vi "Pressures.vi"(7 "Pressure":dbl, 8 "Error In":errorcluster, 9 "File Name In":path, 10 "Interruption Time":dbl, 11 "Flow":dynamicdata(graph)) -> (0 "Error Out":errorcluster, 1 "File Name":path, 2 "Interruption Time":dbl format="%#.3g", 3 "SGP":dbl, 5 "PTP":dbl)   [LabVIEW 2013]
uses:
  Controls/Intervals.ctl
  <vilib>/Utility/miscctls.llb/LVCursorListTypeDef.ctl
  <vilib>/Waveform/WDTOps.llb/WDT Get XY Value DBL.vi
panel:
  in  "Cursor List":T1=[{"Name"="L", "Color"=9843450, "Style"=2, "Point Style"=1, "Name Visible"=FALSE, "Allow Drag"=TRUE, "Cursor Mode"=0, "Plot"=0, "Index"=0, "Position"={"X"=3.0, "Y"=0.0}, "X Scale"=0, "Y Scale"=0, "Watch Plots"=[], "Watch All Plots"=FALSE, "Plot Area"=0, "Label Offset"={"X"=0.0, "Y"=0.0}}, {"Name"="R", "Color"=681210, "Style"=2, "Point Style"=1, "Name Visible"=FALSE, "Allow Drag"=TRUE, "Cursor Mode"=0, "Plot"=0, "Index"=0, "Position"={"X"=3.5, "Y"=0.0}, "X Scale"=0, "Y Scale"=0, "Watch Plots"=[], "Watch All Plots"=FALSE, "Plot Area"=0, "Label Offset"={"X"=0.0, "Y"=0.0}}]
  out "Subset":dynamicdata(graph)
  out "Flow":dynamicdata(graph)
  in  "Interval (ms)":T2 items=["1000", "500", "330", "250", "150", "50"]
  in  "Fixed Length?":bool
  in  "Mark Flow":bool
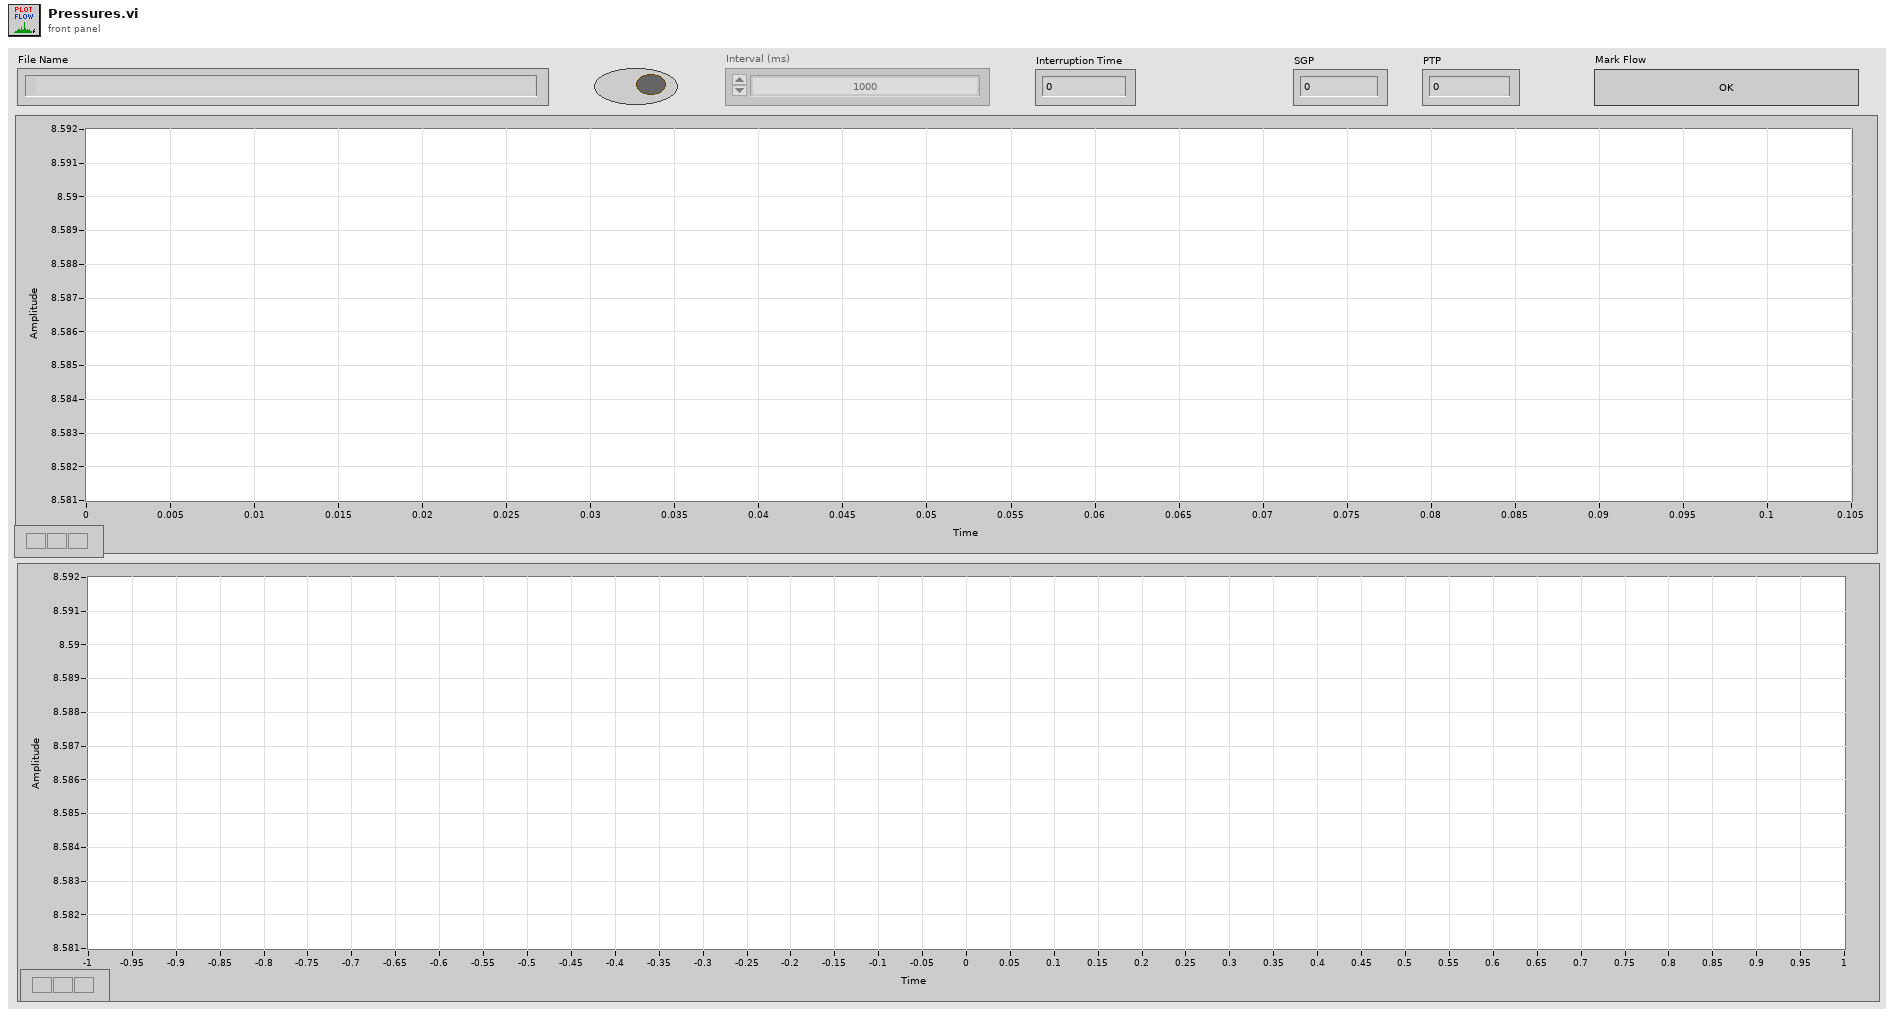
[diagram p1: front panel]
types:
  T1 = typedef "LVCursorListTypeDef.ctl" = cluster{"Name":string, "Color":u32, "Style":u8, "Point Style":u8, "Name Visible":bool, "Allow Drag":bool, "Cursor Mode":u32, "Plot":i32, "Index":i32, "Position":cluster{"X":dbl, "Y":dbl}, "X Scale":u32, "Y Scale":u32, "Watch Plots":i32[], "Watch All Plots":bool, "Plot Area":i32, "Label Offset":cluster{"X":dbl, "Y":dbl}}[]
  T2 = typedef "Intervals.ctl" = u16
  T3 = enum8{"Enabled", "Disabled", "Disabled and Grayed Out"}
  T4 = cluster{"Cursor List[0]":cluster{"Name":string, "Color":u32, "Style":u8, "Point Style":u8, "Name Visible":bool, "Allow Drag":bool, "Cursor Mode":u32, "Plot":i32, "Index":i32, "Position":cluster{"X":dbl, "Y":dbl}, "X Scale":u32, "Y Scale":u32, "Watch Plots":i32[], "Watch All Plots":bool, "Plot Area":i32, "Label Offset":cluster{"X":dbl, "Y":dbl}}, "Cursor List[1]":cluster{"Name":string, "Color":u32, "Style":u8, "Point Style":u8, "Name Visible":bool, "Allow Drag":bool, "Cursor Mode":u32, "Plot":i32, "Index":i32, "Position":cluster{"X":dbl, "Y":dbl}, "X Scale":u32, "Y Scale":u32, "Watch Plots":i32[], "Watch All Plots":bool, "Plot Area":i32, "Label Offset":cluster{"X":dbl, "Y":dbl}}, "Cursor List[2]":cluster{"Name":string, "Color":u32, "Style":u8, "Point Style":u8, "Name Visible":bool, "Allow Drag":bool, "Cursor Mode":u32, "Plot":i32, "Index":i32, "Position":cluster{"X":dbl, "Y":dbl}, "X Scale":u32, "Y Scale":u32, "Watch Plots":i32[], "Watch All Plots":bool, "Plot Area":i32, "Label Offset":cluster{"X":dbl, "Y":dbl}}, "Cursor List[3]":cluster{"Name":string, "Color":u32, "Style":u8, "Point Style":u8, "Name Visible":bool, "Allow Drag":bool, "Cursor Mode":u32, "Plot":i32, "Index":i32, "Position":cluster{"X":dbl, "Y":dbl}, "X Scale":u32, "Y Scale":u32, "Watch Plots":i32[], "Watch All Plots":bool, "Plot Area":i32, "Label Offset":cluster{"X":dbl, "Y":dbl}}, "Cursor List[4]":cluster{"Name":string, "Color":u32, "Style":u8, "Point Style":u8, "Name Visible":bool, "Allow Drag":bool, "Cursor Mode":u32, "Plot":i32, "Index":i32, "Position":cluster{"X":dbl, "Y":dbl}, "X Scale":u32, "Y Scale":u32, "Watch Plots":i32[], "Watch All Plots":bool, "Plot Area":i32, "Label Offset":cluster{"X":dbl, "Y":dbl}}, "Cursor List[5]":cluster{"Name":string, "Color":u32, "Style":u8, "Point Style":u8, "Name Visible":bool, "Allow Drag":bool, "Cursor Mode":u32, "Plot":i32, "Index":i32, "Position":cluster{"X":dbl, "Y":dbl}, "X Scale":u32, "Y Scale":u32, "Watch Plots":i32[], "Watch All Plots":bool, "Plot Area":i32, "Label Offset":cluster{"X":dbl, "Y":dbl}}, "Cursor List[6]":cluster{"Name":string, "Color":u32, "Style":u8, "Point Style":u8, "Name Visible":bool, "Allow Drag":bool, "Cursor Mode":u32, "Plot":i32, "Index":i32, "Position":cluster{"X":dbl, "Y":dbl}, "X Scale":u32, "Y Scale":u32, "Watch Plots":i32[], "Watch All Plots":bool, "Plot Area":i32, "Label Offset":cluster{"X":dbl, "Y":dbl}}, "Cursor List[7]":cluster{"Name":string, "Color":u32, "Style":u8, "Point Style":u8, "Name Visible":bool, "Allow Drag":bool, "Cursor Mode":u32, "Plot":i32, "Index":i32, "Position":cluster{"X":dbl, "Y":dbl}, "X Scale":u32, "Y Scale":u32, "Watch Plots":i32[], "Watch All Plots":bool, "Plot Area":i32, "Label Offset":cluster{"X":dbl, "Y":dbl}}, "Cursor List[8]":cluster{"Name":string, "Color":u32, "Style":u8, "Point Style":u8, "Name Visible":bool, "Allow Drag":bool, "Cursor Mode":u32, "Plot":i32, "Index":i32, "Position":cluster{"X":dbl, "Y":dbl}, "X Scale":u32, "Y Scale":u32, "Watch Plots":i32[], "Watch All Plots":bool, "Plot Area":i32, "Label Offset":cluster{"X":dbl, "Y":dbl}}}
  T5 = cluster{"Name":string, "Color":u32, "Style":u8, "Point Style":u8, "Name Visible":bool, "Allow Drag":bool, "Cursor Mode":u32, "Plot":i32, "Index":i32, "Position":cluster{"X":dbl, "Y":dbl}, "X Scale":u32, "Y Scale":u32, "Watch Plots":i32[], "Watch All Plots":bool, "Plot Area":i32, "Label Offset":cluster{"X":dbl, "Y":dbl}}[]
  T6 = cluster{"CrsrList[0]":cluster{"Name":string, "Color":u32, "Style":u8, "Point Style":u8, "Name Visible":bool, "Allow Drag":bool, "Cursor Mode":u32, "Plot":i32, "Index":i32, "Position":cluster{"X":dbl, "Y":dbl}, "X Scale":u32, "Y Scale":u32, "Watch Plots":i32[], "Watch All Plots":bool, "Plot Area":i32, "Label Offset":cluster{"X":dbl, "Y":dbl}}, "CrsrList[1]":cluster{"Name":string, "Color":u32, "Style":u8, "Point Style":u8, "Name Visible":bool, "Allow Drag":bool, "Cursor Mode":u32, "Plot":i32, "Index":i32, "Position":cluster{"X":dbl, "Y":dbl}, "X Scale":u32, "Y Scale":u32, "Watch Plots":i32[], "Watch All Plots":bool, "Plot Area":i32, "Label Offset":cluster{"X":dbl, "Y":dbl}}, "CrsrList[2]":cluster{"Name":string, "Color":u32, "Style":u8, "Point Style":u8, "Name Visible":bool, "Allow Drag":bool, "Cursor Mode":u32, "Plot":i32, "Index":i32, "Position":cluster{"X":dbl, "Y":dbl}, "X Scale":u32, "Y Scale":u32, "Watch Plots":i32[], "Watch All Plots":bool, "Plot Area":i32, "Label Offset":cluster{"X":dbl, "Y":dbl}}, "CrsrList[3]":cluster{"Name":string, "Color":u32, "Style":u8, "Point Style":u8, "Name Visible":bool, "Allow Drag":bool, "Cursor Mode":u32, "Plot":i32, "Index":i32, "Position":cluster{"X":dbl, "Y":dbl}, "X Scale":u32, "Y Scale":u32, "Watch Plots":i32[], "Watch All Plots":bool, "Plot Area":i32, "Label Offset":cluster{"X":dbl, "Y":dbl}}, "CrsrList[4]":cluster{"Name":string, "Color":u32, "Style":u8, "Point Style":u8, "Name Visible":bool, "Allow Drag":bool, "Cursor Mode":u32, "Plot":i32, "Index":i32, "Position":cluster{"X":dbl, "Y":dbl}, "X Scale":u32, "Y Scale":u32, "Watch Plots":i32[], "Watch All Plots":bool, "Plot Area":i32, "Label Offset":cluster{"X":dbl, "Y":dbl}}, "CrsrList[5]":cluster{"Name":string, "Color":u32, "Style":u8, "Point Style":u8, "Name Visible":bool, "Allow Drag":bool, "Cursor Mode":u32, "Plot":i32, "Index":i32, "Position":cluster{"X":dbl, "Y":dbl}, "X Scale":u32, "Y Scale":u32, "Watch Plots":i32[], "Watch All Plots":bool, "Plot Area":i32, "Label Offset":cluster{"X":dbl, "Y":dbl}}, "CrsrList[6]":cluster{"Name":string, "Color":u32, "Style":u8, "Point Style":u8, "Name Visible":bool, "Allow Drag":bool, "Cursor Mode":u32, "Plot":i32, "Index":i32, "Position":cluster{"X":dbl, "Y":dbl}, "X Scale":u32, "Y Scale":u32, "Watch Plots":i32[], "Watch All Plots":bool, "Plot Area":i32, "Label Offset":cluster{"X":dbl, "Y":dbl}}, "CrsrList[7]":cluster{"Name":string, "Color":u32, "Style":u8, "Point Style":u8, "Name Visible":bool, "Allow Drag":bool, "Cursor Mode":u32, "Plot":i32, "Index":i32, "Position":cluster{"X":dbl, "Y":dbl}, "X Scale":u32, "Y Scale":u32, "Watch Plots":i32[], "Watch All Plots":bool, "Plot Area":i32, "Label Offset":cluster{"X":dbl, "Y":dbl}}, "CrsrList[8]":cluster{"Name":string, "Color":u32, "Style":u8, "Point Style":u8, "Name Visible":bool, "Allow Drag":bool, "Cursor Mode":u32, "Plot":i32, "Index":i32, "Position":cluster{"X":dbl, "Y":dbl}, "X Scale":u32, "Y Scale":u32, "Watch Plots":i32[], "Watch All Plots":bool, "Plot Area":i32, "Label Offset":cluster{"X":dbl, "Y":dbl}}}
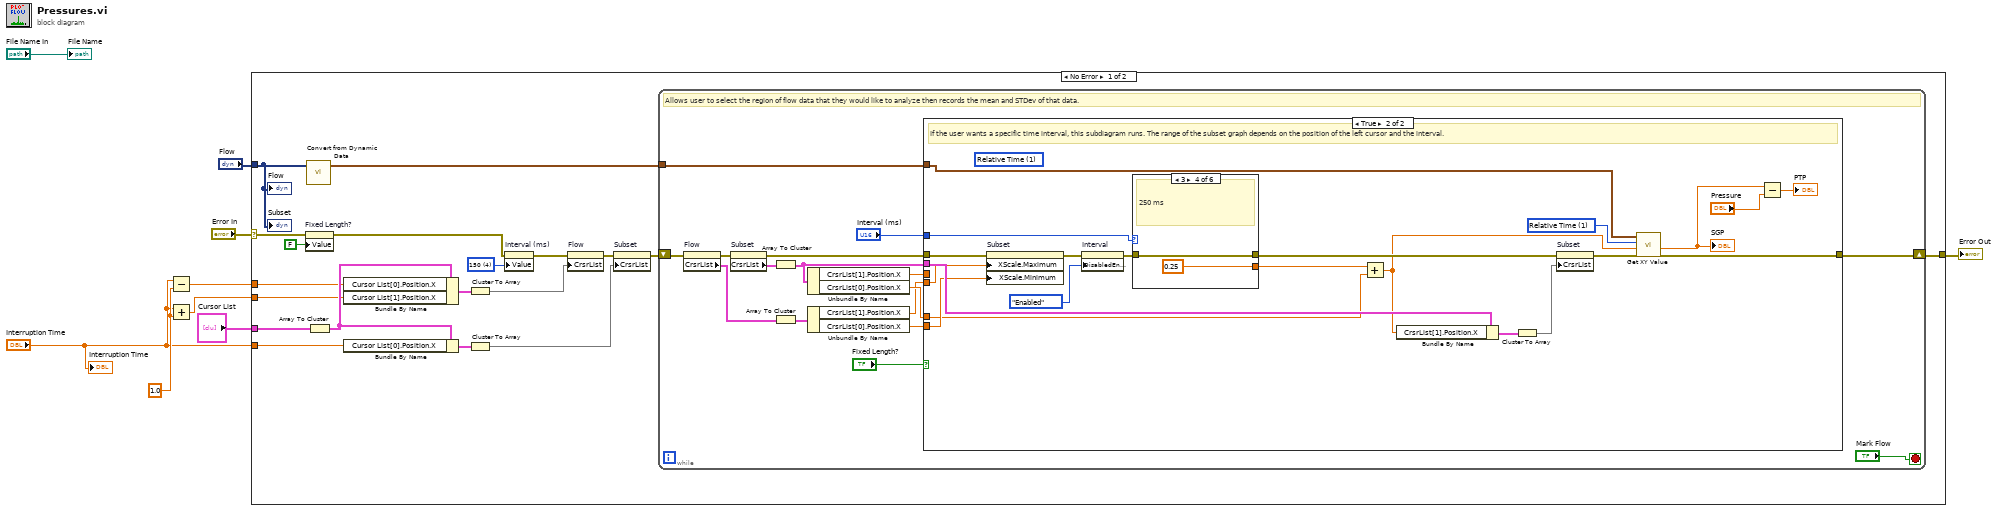
[diagram p0: block diagram]
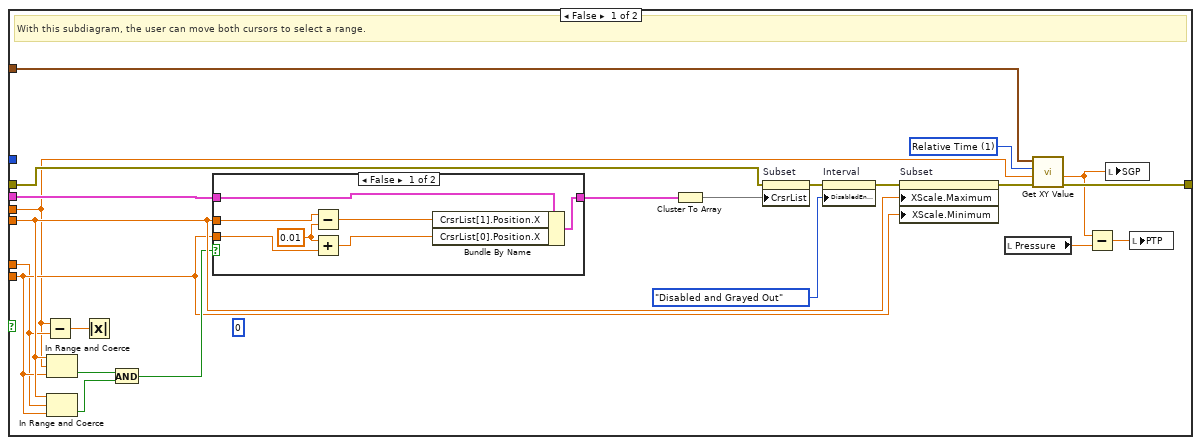
[diagram p2: hidden frame]
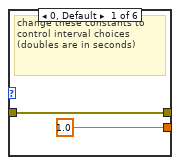
[diagram p4: hidden frame]
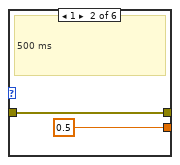
[diagram p5: hidden frame]
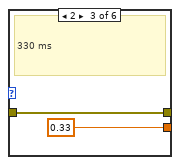
[diagram p6: hidden frame]
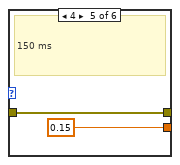
[diagram p7: hidden frame]
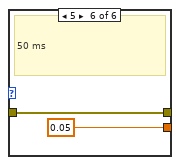
[diagram p8: hidden frame]
diagram:
  w3 = 1.0 ("y")
  n1 = Subtract(x="Interruption Time", y=w3) -> (x-y=w2:dbl)
  n2 = Add(x="Interruption Time", y=w3) -> (x+y=w4:dbl)
  n3 = case shown="No Error" "Error In" {
    selector: "Error In" -> [w20 w108]
    tunnel: "Flow" -> [w27 _]
    tunnel: [w28 w108] -> w6
    tunnel: "Interruption Time" -> [w23 _]
    tunnel: "Cursor List" -> [w24 _]
    tunnel: w4 -> [w12 _]
    tunnel: w2 -> [w11 _]
    frame No Error {
      w18 = T2 4 items=["1000", "500", "330", "250", "150", "50"] ("Interval (ms)")
      n4 = property on="Fixed Length?" class="Bool (strict)"(error in=w20, "Value"=FALSE ("Fixed Length?")) -> (error out=w10:errorcluster)  [unwired: 1 in, 1 out]
      n5 = call "Convert from Dynamic Data"("Dynamic Data Type"=w27) -> ("Waveform"=w26:waveform(dbl))  [unwired: 3 in]
      n6 = Array To Cluster(array=w24) -> (cluster=w15:T4)
      n7 = Bundle By Name(cluster=w15, "Cursor List[0].Position.X"=w11, "Cursor List[1].Position.X"=w12) -> (w14:T4)
      n8 = Bundle By Name(cluster=w15, "Cursor List[0].Position.X"=w23) -> (w22:T4)
      n9 = Cluster To Array(cluster=w14) -> (array=w13:T5)
      n10 = Cluster To Array(cluster=w22) -> (array=w21:T5)
      n11 = property on="Interval (ms)" class="Ring (strict)"(error in=w10, "Value"=w18) -> (error out=w17:errorcluster)  [unwired: 1 in, 1 out]
      n12 = property on="Flow" class="WFGraph (strict)"(error in=w17, "CrsrList"=w13) -> (error out=w16:errorcluster)  [unwired: 1 in, 1 out]
      n13 = property on="Subset" class="WFGraph (strict)"(error in=w16, "CrsrList"=w21) -> (error out=w25:errorcluster)  [unwired: 1 in, 1 out]
      n14 = while {
        shift-right: [w41] -> w28
        shift-left: w25 -> [w39]
        tunnel: w26 -> [w32]
        stop <- "Mark Flow" stop-if-true
        # "Allows user to select the region of flow data that they would like to analyze then records the mean and STDev of that data."
        n15 = property on="Flow" class="WFGraph (strict)"(error in=w39) -> (error out=w37:errorcluster, "CrsrList"=w38:T1)  [unwired: 1 in, 1 out]
        n16 = property on="Subset" class="WFGraph (strict)"(error in=w37) -> (error out=w29:errorcluster, "CrsrList"=w36:T1)  [unwired: 1 in, 1 out]
        n17 = Array To Cluster(array=w36) -> (cluster=w33:T6)
        n18 = Array To Cluster(array=w38) -> (cluster=w40:T6)
        n19 = Unbundle By Name(w33) -> ("CrsrList[1].Position.X"=w34:dbl, "CrsrList[0].Position.X"=w35:dbl)
        n20 = Unbundle By Name(w40) -> ("CrsrList[1].Position.X"=w31:dbl, "CrsrList[0].Position.X"=w30:dbl)
        n21 = case shown="True" "Fixed Length?" {
          tunnel: "Interval (ms)" -> [_ w94]
          tunnel: [w48 w80] -> w41
          tunnel: w31 -> [w61 w87]
          tunnel: w30 -> [w56 w86]
          tunnel: w32 -> [w51 w82]
          tunnel: w34 -> [w49 _]
          tunnel: w35 -> [w54 w83]
          tunnel: w33 -> [w64 w91]
          tunnel: w29 -> [w53 w85]
          frame False {
            (unwired) 0 ("Start Index")
            w50 = u16 1 items=["Samples", "Relative Time"] ("start/duration format")
            # "With this subdiagram, the user can move both cursors to select a range."
            n22 = Subtract(x=w49, y=w54) -> (x-y=w55:dbl)
            n23 = In Range and Coerce(upper limit=w61, x=w49, lower limit=w56) -> (In Range?=w59:bool)  [unwired: 1 out]
            n24 = In Range and Coerce(upper limit=w61, x=w54, lower limit=w56) -> (In Range?=w58:bool)  [unwired: 1 out]
            n25 = Absolute Value(x=w55) -> ()  [unwired: 1 out]
            n26 = And(x=w59, y=w58) -> (x .and. y?=w57:bool)
            n27 = case shown="False" w57 {
              tunnel: w64 -> [w73 w74]
              tunnel: [w72 w74] -> w62
              tunnel: w61 -> [w70 _]
              tunnel: w56 -> [w69 _]
              frame False {
                w67 = 0.01 ("y")
                # "Right Cursor"
                n28 = Subtract(x=w70, y=w67) -> (x-y=w71:dbl)
                n29 = Add(x=w67, y=w69) -> (x+y=w68:dbl)
                n30 = Bundle By Name(cluster=w73, "CrsrList[1].Position.X"=w71, "CrsrList[0].Position.X"=w68) -> (w72:T6)
              }
              frame True {
                # "Right Cursor"
              }
            }
            n31 = Cluster To Array(cluster=w62) -> (array=w63:T5)
            n32 = property on="Subset" class="WFGraph (strict)"(error in=w53, "CrsrList"=w63) -> (error out=w60:errorcluster)  [unwired: 1 in, 1 out]
            n33 = property on="Interval" class="Ring (strict)"(error in=w60, "DisabledEnum"=T3."Disabled and Grayed Out" ("Disabled")) -> (error out=w65:errorcluster)  [unwired: 1 in, 1 out]
            n34 = property on="Subset" class="WFGraph (strict)"(error in=w65, "XScale.Maximum"=w61, "XScale.Minimum"=w56) -> (error out=w52:errorcluster)  [unwired: 1 in, 1 out]
            n35 = local read "Pressure"() -> (w47:dbl)
            n36 = call-poly <vilib>:"Get XY Value.vi"("error in (no error)"=w52, "Y position"=w49, "Y position format"=w50, "waveform in"=w51) -> ("error out"=w48:errorcluster, "Y value"=w46:dbl)  [unwired: 3 in, 3 out]
            n37 = Subtract(x=w46, y=w47) -> (x-y=w45:dbl)
            n38 = local write "SGP"(w46) -> ()
            n39 = local write "PTP"(w45) -> ()
          }
          frame True {
            w76 = u16 1 items=["Samples", "Relative Time"] ("Y position format")
            (unwired) u16 1 items=["Samples", "Relative Time"] ("start/duration format")
            # "If the user wants a specific time interval, this subdiagram runs. The range of the subset graph depends on the position of the left cursor and the interval."
            n40 = property on="Subset" class="WFGraph (strict)"(error in=w85, "XScale.Maximum"=w87, "XScale.Minimum"=w86) -> (error out=w84:errorcluster)  [unwired: 1 in, 1 out]
            n41 = property on="Interval" class="Ring (strict)"(error in=w84, "DisabledEnum"=T3."Enabled" ("Disabled")) -> (error out=w93:errorcluster)  [unwired: 1 in, 1 out]
            n42 = case shown="3" w94 {
              tunnel: [w97 w99 w101 w103 w105 w107] -> w88
              tunnel: w93 -> [w97 w99 w101 w103 w105 w107]
              tunnel: [1.0 ("CrsrList[0].Position.X") 0.5 ("CrsrList[0].Position.X") 0.33 ("CrsrList[0].Position.X") 0.25 ("CrsrList[0].Position.X") 0.15 ("CrsrList[0].Position.X") 0.05 ("CrsrList[0].Position.X")] -> w92
              frame 0, Default {
                # "change these constants to control interval choices (doubles are in seconds)"
              }
              frame 1 {
                # "500 ms"
              }
              frame 2 {
                # "330 ms"
              }
              frame 3 {
                # "250 ms"
              }
              frame 4 {
                # "150 ms"
              }
              frame 5 {
                # "50 ms"
              }
            }
            n43 = Add(x=w92, y=w83) -> (x+y=w79:dbl)
            n44 = Bundle By Name(cluster=w91, "CrsrList[1].Position.X"=w79) -> (w89:T6)
            n45 = Cluster To Array(cluster=w89) -> (array=w90:T5)
            n46 = property on="Subset" class="WFGraph (strict)"(error in=w88, "CrsrList"=w90) -> (error out=w81:errorcluster)  [unwired: 1 in, 1 out]
            n47 = call-poly <vilib>:"Get XY Value.vi"("error in (no error)"=w81, "Y position"=w79, "Y position format"=w76, "waveform in"=w82) -> ("error out"=w80:errorcluster, "Y value"=w78:dbl)  [unwired: 3 in, 3 out]
            "SGP" <- w78
            n48 = Subtract(x=w78, y="Pressure") -> (x-y=→"PTP":dbl)
          }
        }
      }
      "Flow" <- w27
      "Subset" <- w27
    }
    frame Error {
    }
  }
  "Error Out" <- w6
  "File Name" <- "File Name In"
  "Interruption Time" <- "Interruption Time"
